vi "Simple Example for Docs.vi"() -> ()   [LabVIEW 2018]
uses:
  api/Failure Information.ctl
  api/Log Record.ctl
  api/logger_class/Internal Log Levels.ctl
  4be55814-5d04-44e5-93a4-e1fe601a205d.vi
  11498d54-b0da-4181-bfbd-37c405b816d5.vi
  0679c0b6-e665-4267-8d21-5c2f63ff0cfc.vi
  b68c178a-45ff-4a43-8ee1-f997d7190e6c.vi
  26cdefab-9c11-46d6-bea8-26d872e8373c.vi
  cd3cbcb6-eea4-4d7a-90d3-75033959401d.vi
  3aace37d-2631-4088-b4d1-fd5fc03c86bc.vi
  4be55814-5d04-44e5-93a4-e1fe601a205d.vi/1f4baa75-7c2a-40e9-b4bc-d287912a8f57.vi
  11498d54-b0da-4181-bfbd-37c405b816d5.vi/28727e37-b0d9-407c-a479-ab0b7779cd69.vi
  0679c0b6-e665-4267-8d21-5c2f63ff0cfc.vi/a153a250-4fb8-4a99-bb5b-6ccb57f1f631.vi
  b68c178a-45ff-4a43-8ee1-f997d7190e6c.vi/a02c6254-97f5-44e3-a3a9-7fdb6dfbd055.vi
  26cdefab-9c11-46d6-bea8-26d872e8373c.vi/bae24b8d-f663-491e-8374-2218e527d0d0.vi
  cd3cbcb6-eea4-4d7a-90d3-75033959401d.vi/bf655d3c-1ce4-400f-a78f-0f3f0191886e.vi
  api/Mark Error.vi
  3aace37d-2631-4088-b4d1-fd5fc03c86bc.vi/ba94d47b-0e30-4c32-b8ff-86d609cd95a5.vi
  0679c0b6-e665-4267-8d21-5c2f63ff0cfc.vi/a153a250-4fb8-4a99-bb5b-6ccb57f1f631.vi/28727e37-b0d9-407c-a479-ab0b7779cd69.vi
  b68c178a-45ff-4a43-8ee1-f997d7190e6c.vi/a02c6254-97f5-44e3-a3a9-7fdb6dfbd055.vi/7453dcce-b283-4a0d-ab92-51c518b086c4.vi
  26cdefab-9c11-46d6-bea8-26d872e8373c.vi/bae24b8d-f663-491e-8374-2218e527d0d0.vi/083db1d9-8cf1-45e4-a540-e8e178cc7cc8.vi
  registry/Log.vi
  api/Logging.lvlib
panel:
  in  "abort":bool
  in  "path (use dialog)":path[](array[path])
  out "failures info":T1[](array[typedef]) {"Log Record"."timestamp" format="%<%x %.3X>T"}
  out "error out":errorcluster
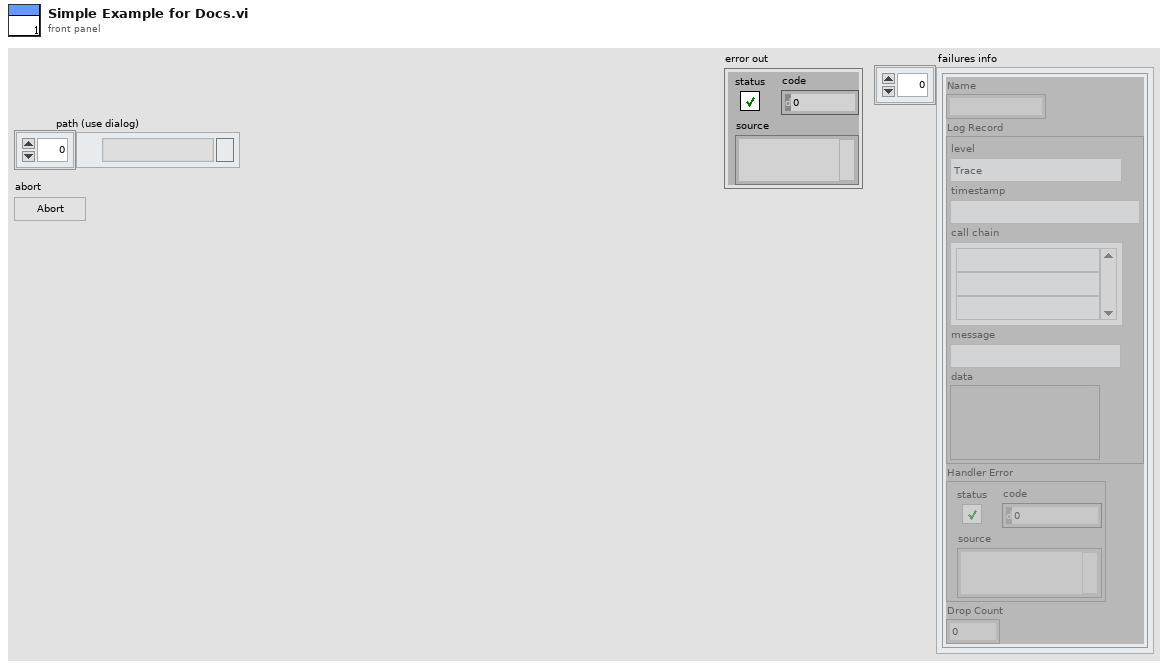
[diagram p1: front panel]
types:
  T1 = typedef "Logging.lvlib/Failure Information.ctl" = cluster{"Name":string, "Log Record":T2, "Handler Error":errorcluster, "Drop Count":u32}
  T2 = typedef "Logging.lvlib/Log Record.ctl" = cluster{"level":T3, "timestamp":timestamp, "call chain":string[], "message":string, "data":variant}
  T3 = typedef "Logging.lvlib/Internal Log Levels.ctl" = enum16{"Trace", "Debug", "Info", "Warning", "Error", "Critical", "Internal"}
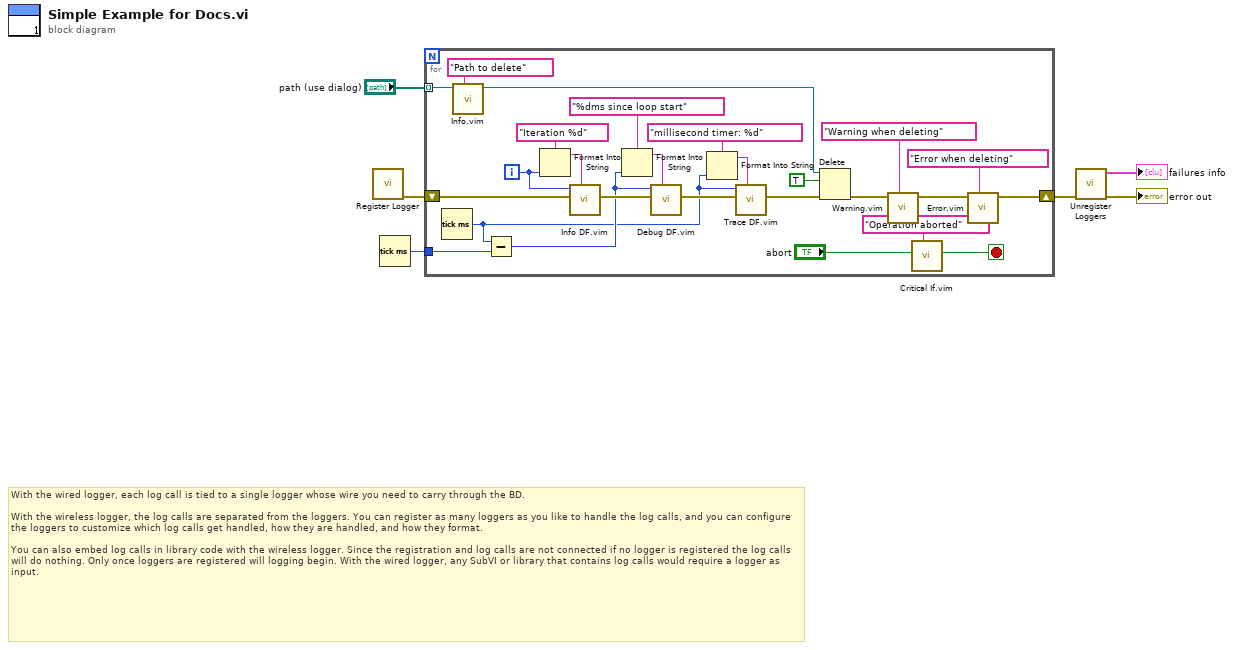
[diagram p0: block diagram]
diagram:
  # "With the wired logger, each log call is tied to a single logger whose wire you need to carry through the BD.\n\nWith the wireless logger, the log calls are separated from the loggers. You can register as many loggers as you like to handle the log calls, and you can configure the loggers to customize which log calls get handled, how they are handled, and how they format.\n\nYou can also embed log calls in library code with the wireless logger. Since the registration and log calls are not connected if no logger is registered the log calls will do nothing. Only once loggers are registered will logging begin. With the wired logger, any SubVI or library that contains log calls would require a logger as input."
  n1 = call "Register Logger.vi"() -> ("error out"=w2:errorcluster)  [unwired: 11 in]
  n2 = Tick Count (ms)() -> (millisecond timer value=w6:u32)
  n3 = for {
    shift-right: [w21] -> w3
    shift-left: w2 -> [w30]
    tunnel: "path (use dialog)" -> [w14] mode=indexing
    tunnel: w6 -> [w32]
    i -> [w19]
    stop <- w8 stop-if-true
    n4 = Tick Count (ms)() -> (millisecond timer value=w13:u32)
    n5 = call "Info.vim"("data in (null)"=w14, "message"="Path to delete") -> ("data out"=w12:path)  [unwired: 9 in]
    n6 = Subtract(x=w13, y=w32) -> (x-y=w26:u32)
    n7 = Format Into String(format string="Iteration %d" ("message"), w19) -> (resulting string=w29:string)  [unwired: 2 in, 1 out]
    n8 = call "Info DF.vim"("message"=w29, "dataflow in"=w30, "data (null)"=w19) -> ("dataflow out"=w27:errorcluster)  [unwired: 8 in]
    n9 = Format Into String(format string="%dms since loop start" ("message"), w26) -> (resulting string=w28:string)  [unwired: 2 in, 1 out]
    n10 = call "Debug DF.vim"("message"=w28, "dataflow in"=w27, "data (null)"=w26) -> ("dataflow out"=w22:errorcluster)  [unwired: 8 in]
    n11 = Format Into String(format string="millisecond timer: %d" ("message"), w13) -> (resulting string=w23:string)  [unwired: 2 in, 1 out]
    n12 = call "Trace DF.vim"("message"=w23, "dataflow in"=w22, "data (null)"=w13) -> ("dataflow out"=w16:errorcluster)  [unwired: 8 in]
    n13 = Delete(path (use dialog)=w12, entire hierarchy (F)=TRUE, error in=w16) -> (error out=w15:errorcluster)  [unwired: 2 in, 2 out]
    n14 = call "Warning.vim"("data in (null)"=w15, "message"="Warning when deleting") -> ("data out"=w18:errorcluster)  [unwired: 9 in]
    n15 = call "Critical If.vim"("message"="Operation aborted", "condition in"="abort") -> ("condition out"=w8:bool)  [unwired: 9 in]
    n16 = call "Error.vim"("data in (null)"=w18, "message"="Error when deleting") -> ("data out"=w21:errorcluster)  [unwired: 9 in]
  }
  n17 = call "Unregister Loggers.vi"("error in (no error)"=w3) -> ("error out"=→"error out":errorcluster, "failures info"=→"failures info":T1[])  [unwired: 9 in]
